vi "IntensityGraphFFT.vi"(0 "Data In":T6={"Cluster"={"2^n : x"=1, "2^n : y"=1, "lower left box Position"={"X"=0.0, "Y"=0.0}}, "Array"=[]} {"Cluster"."2^n : y" min=1 max=13; "Cluster"."2^n : x" min=1 max=13}, 2 "Display State In":T4, 3 "Container State":T5) -> (6 "Data Out":T6={"Cluster"={"2^n : x"=1, "2^n : y"=1, "lower left box Position"={"X"=0.0, "Y"=0.0}}, "Array"=[]} {"Cluster"."2^n : y" min=1 max=13; "Cluster"."2^n : x" min=1 max=13}, 7 "Display State Out":T4, 8 "Action":T3)   [LabVIEW 2018, in "XControl 1.xctl"]
uses:
  XControl 1.xctl
  2Ddatas.ctl
  <vilib>/Utility/miscctls.llb/LVPointDoubleTypeDef.ctl
  <vilib>/_xctls/Container State.ctl
  State 1.ctl
  <vilib>/_xctls/Action.ctl
  <vilib>/_xctls/XControlSupport.lvlib
panel:
  in  "Cluster":T2={"2^n : x"=1, "2^n : y"=1, "lower left box Position"={"X"=0.0, "Y"=0.0}} {"2^n : y" min=1 max=13; "2^n : x" min=1 max=13}
  out "output FFT \ndimension":T1
  out "Intensity Graph":dbl[][](graph)
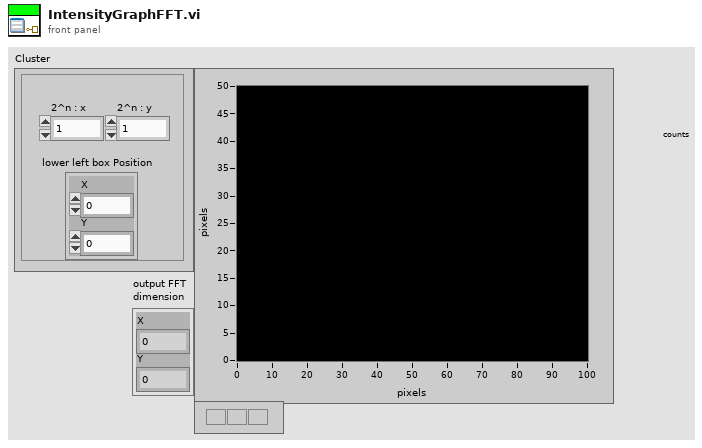
[diagram p1: front panel]
types:
  T1 = typedef "LVPointDoubleTypeDef.ctl" = cluster{"X":dbl, "Y":dbl}
  T2 = cluster{"2^n : x":i8, "2^n : y":i8, "lower left box Position":T1}
  T3 = typedef "XControlSupport.lvlib/Action.ctl" = cluster{"Data Changed?":bool, "State Changed?":bool, "Action Name":string}
  T4 = typedef "XControl 1.xctl/State 1.ctl" = cluster{"Numeric":dbl}
  T5 = typedef "XControlSupport.lvlib/Container State.ctl" = cluster{"Indicator?":bool, "Run Mode?":bool, " Refnum":refnum<vi>}
  T6 = typedef "XControl 1.xctl/2Ddatas.ctl" = cluster{"Cluster":cluster{"2^n : x":i8, "2^n : y":i8, "lower left box Position":T1}, "Array":dbl[][]}
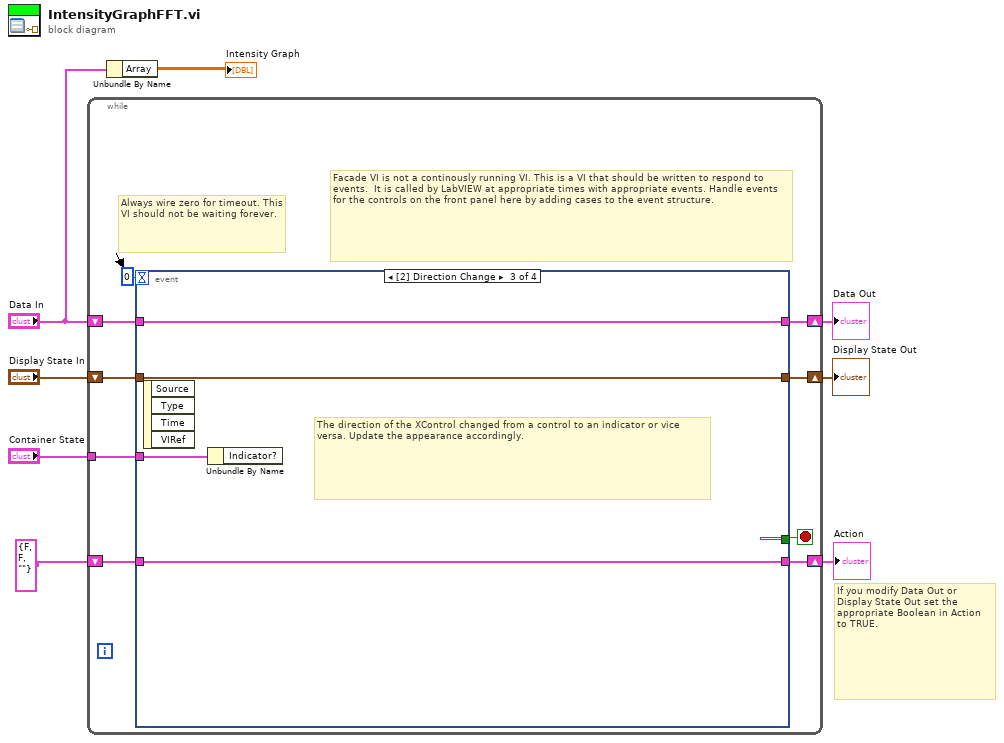
[diagram p0: block diagram]
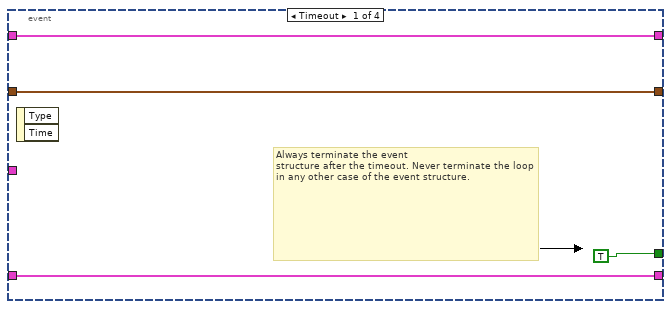
[diagram p2: hidden frame]
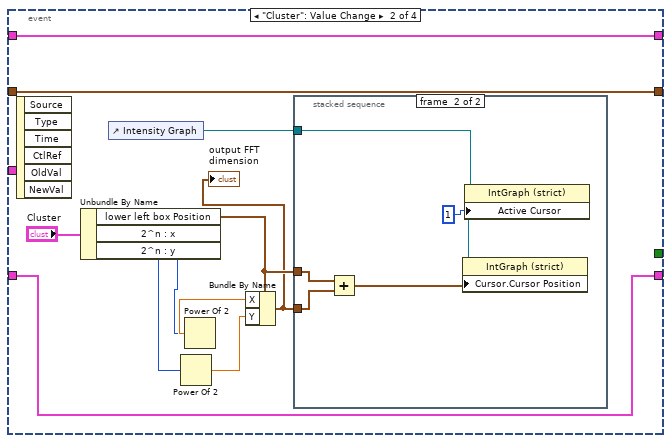
[diagram p3: hidden frame]
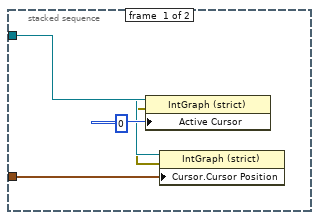
[diagram p4: hidden frame]
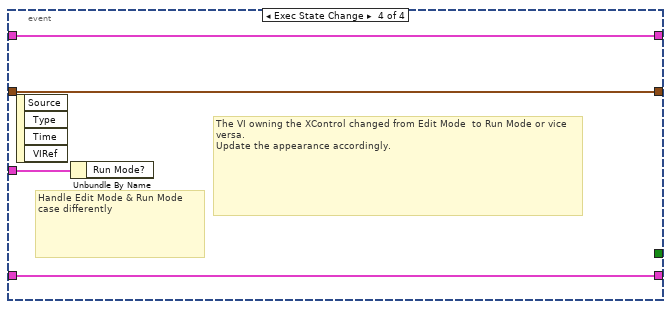
[diagram p5: hidden frame]
diagram:
  # "If you modify Data Out or\nDisplay State Out set the\nappropriate Boolean in Action\nto TRUE."
  n1 = while {
    shift-right: [w16] -> w6
    shift-left: "Display State In" -> [w17]
    tunnel: "Container State" -> [w13]
    shift-right: [w12] -> w8
    shift-left: "Data In" -> [w9]
    shift-right: [w10] -> w4
    shift-left: T3 {"Data Changed?"=FALSE, "State Changed?"=FALSE, "Action Name"=""} ("Action") -> [w11]
    stop <- w15 stop-if-true
    # "Facade VI is not a continously running VI. This is a VI that should be written to respond to events.  It is called by LabVIEW at appropriate times with appropriate events. Handle events for the controls on the front panel here by adding cases to the event structure."
    # "Always wire zero for timeout. This\nVI should not be waiting forever."
    n2 = event shown="[2] Direction Change" {
      selector: _ -> [_ _ _ _]
      dyn-events: _ -> [_ _ _ _]
      timeout: 0 -> [_ _ _ _]
      tunnel: w17 -> [w19 w32 w47 w51]
      tunnel: [w19 w32 w47 w51] -> w16
      tunnel: [TRUE _ _ _] -> w15
      tunnel: w13 -> [_ _ w48 w52]
      tunnel: w9 -> [w18 w31 w46 w50]
      tunnel: [w18 w31 w46 w50] -> w12
      tunnel: [w20 w30 w45 w49] -> w10
      tunnel: w11 -> [w20 w30 w45 w49]
      event Timeout {
        # "Always terminate the event\nstructure after the timeout. Never terminate the loop in any other case of the event structure."
        n3 = event-data() -> ()  [unwired: 1 in, 2 out]
      }
      event "Cluster": Value Change {
        n4 = event-data() -> ()  [unwired: 1 in, 6 out]
        n5 = Unbundle By Name("Cluster") -> ("lower left box Position"=w24:T1, "2^n : x"=w25:i8, "2^n : y"=w26:i8)
        n6 = control-ref of="Intensity Graph"() -> (w29:refnum<vi>)
        n7 = Power Of 2(x=w26) -> (2^x=w27:dbl)
        n8 = Power Of 2(x=w25) -> (2^x=w28:dbl)
        n9 = Bundle By Name(cluster=w24, "X"=w28, "Y"=w27) -> (w23:T1)
        "output FFT \ndimension" <- w23
        n10 = stacked-sequence {
          tunnel: w29 -> [w36 w44]
          tunnel: w24 -> [w33 w40]
          tunnel: w23 -> [_ w39]
          frame #0 {
            n11 = property class="IntGraph (strict)"(reference=w36, "Active Cursor"=u32 0) -> (reference out=w35:refnum<vi>, error out=w34:errorcluster)  [unwired: 1 in]
            n12 = property class="IntGraph (strict)"(reference=w35, error in=w34, "Cursor.Cursor Position"=w33) -> ()  [unwired: 2 out]
          }
          frame #1 {
            n13 = Add(x=w40, y=w39) -> (x+y=w38:T1)
            n14 = property class="IntGraph (strict)"(reference=w44, "Active Cursor"=u32 1) -> (reference out=w42:refnum<vi>, error out=w41:errorcluster)  [unwired: 1 in]
            n15 = property class="IntGraph (strict)"(reference=w42, error in=w41, "Cursor.Cursor Position"=w38) -> ()  [unwired: 2 out]
          }
        }
      }
      event Direction Change {
        # "The direction of the XControl changed from a control to an indicator or vice versa. Update the appearance accordingly."
        n16 = event-data() -> ()  [unwired: 1 in, 4 out]
        n17 = Unbundle By Name(w48) -> ()  [unwired: 1 out]
      }
      event Exec State Change {
        # "The VI owning the XControl changed from Edit Mode  to Run Mode or vice versa.\nUpdate the appearance accordingly."
        # "Handle Edit Mode & Run Mode\ncase differently"
        n18 = event-data() -> ()  [unwired: 1 in, 4 out]
        n19 = Unbundle By Name(w52) -> ()  [unwired: 1 out]
      }
    }
  }
  "Display State Out" <- w6
  "Data Out" <- w8
  "Action" <- w4
  n20 = Unbundle By Name("Data In") -> ("Array"=→"Intensity Graph":dbl[][])
